vi "saveDataNodeBegin.vi"(8 "error in (no error)":errorcluster, 9 "indent":i32, 10 "XML Refnum in":refnum<file>, 11 "Channel_FXP in":refnum<class "Channel_FXP.lvclass">) -> (0 "error out":errorcluster, 2 "XML Refnum out":refnum<file>, 3 "Chennel out":refnum<class "Channel_FXP.lvclass">)   [LabVIEW 2013, in "Channel_FXP.lvclass"]
doc: "Begins the process of saving a xceData Node to an XML formatted file."
uses:
  Channel_FXP.lvclass
  Channel/Channel.lvclass
  Channel_FXP.lvclass/Channel_FXP.ctl
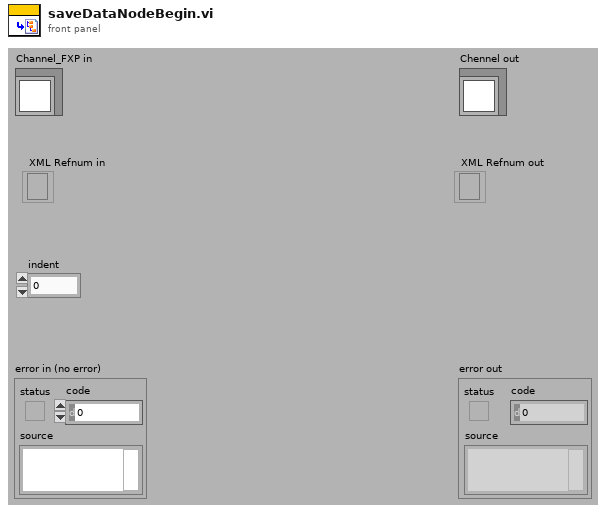
[diagram p1: front panel]
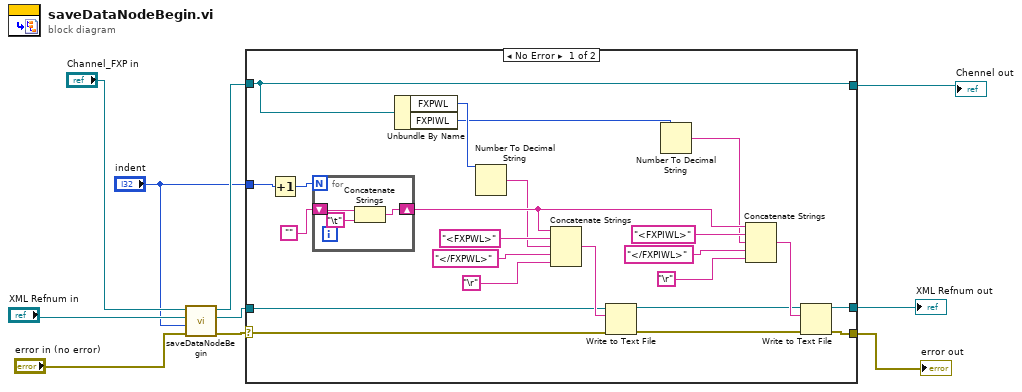
[diagram p0: block diagram]
diagram:
  n1 = call-parent "saveDataNodeBegin.vi"("error in (no error)"="error in (no error)", "indent"="indent", "XML Refnum in"="XML Refnum in", "Channel in"="Channel_FXP in") -> ("error out"=w7:errorcluster, "XML Refnum out"=w4:refnum<file>, "Chennel out"=w5:refnum<class "Channel_FXP.lvclass">)  [unwired: 5 in]
  n2 = case shown="No Error" w7 {
    selector: w7 -> [w17 w38]
    tunnel: w5 -> [w19 w39]
    tunnel: [w19 w39] -> w10
    tunnel: [w27 w38] -> w8
    tunnel: [w29 w37] -> w9
    tunnel: w4 -> [w18 w37]
    tunnel: "indent" -> [w12 _]
    frame No Error {
      n3 = Increment(x=w12) -> (x+1=w11:i32)
      n4 = for {
        N: w11 -> [_]
        shift-right: [w34] -> w22
        shift-left: "" -> [w36]
        n5 = Concatenate Strings(w36, "\t") -> (w34:string)
      }
      n6 = Unbundle By Name(w19) -> ("FXPWL"=w15:i32, "FXPIWL"=w14:i32)
      n7 = Number To Decimal String(number=w15) -> (decimal integer string=w16:string)  [unwired: 1 in]
      n8 = Concatenate Strings(w22, "<FXPWL>" ("string"), w16, "</FXPWL>" ("string"), "\r") -> (w26:string)
      n9 = Write to Text File(file (use dialog)=w18, text=w26, error in=w17) -> (refnum out=w21:refnum<file>, error out=w20:errorcluster)  [unwired: 1 in, 1 out]
      n10 = Number To Decimal String(number=w14) -> (decimal integer string=w13:string)  [unwired: 1 in]
      n11 = Concatenate Strings(w22, "<FXPIWL>" ("string"), w13, "</FXPIWL>" ("string"), "\r") -> (w28:string)
      n12 = Write to Text File(file (use dialog)=w21, text=w28, error in=w20) -> (refnum out=w29:refnum<file>, error out=w27:errorcluster)  [unwired: 1 in, 1 out]
    }
    frame Error {
    }
  }
  "error out" <- w8
  "Chennel out" <- w10
  "XML Refnum out" <- w9
